vi "Gyro.vi"(8 "error in (no error)":errorcluster, 11 "GyroDevRef":T1) -> (1 "Boolean":bool)   [LabVIEW 2013]
uses:
  <vilib>/Rock Robotics/WPI/Gyro/WPI_GyroDevRef.ctl
  <vilib>/Rock Robotics/SystemInterfaces/Typedef/FPGA_TypedefAnalogModule.ctl
  <vilib>/Rock Robotics/SystemInterfaces/AI/FPGA_AIChannel.ctl
  <vilib>/Rock Robotics/WPI/DriverStation/DriverStationLCD/WPI_DriverStationLCDLCDLine.ctl
  Robot Global Data.vi
  <vilib>/Rock Robotics/WPI/Joystick/WPI_JoystickGetSetRefNum.vi
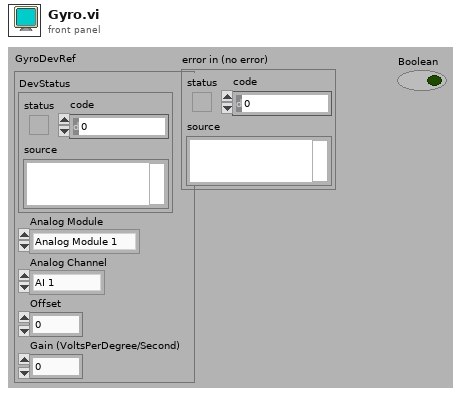
[diagram p1: front panel]
types:
  T1 = typedef "WPI_GyroDevRef.ctl" = cluster{"DevStatus":errorcluster, "Analog Module":T2, "Analog Channel":T3, "Offset":dbl, "Gain (VoltsPerDegree/Second)":dbl}
  T2 = typedef "FPGA_TypedefAnalogModule.ctl" = enum16{"Analog Module 1", "Analog Module 2"}
  T3 = typedef "FPGA_AIChannel.ctl" = enum8{"AI 1", "AI 2", "AI 3", "AI 4", "AI 5", "AI 6", "AI 7", "AI 8", "Invalid"}
  T4 = typedef "WPI_DriverStationLCDLCDLine.ctl" = enum16{"Main - Line 1", "User - Line 2", "User - Line 3", "User - Line 4", "User - Line 5", "User - Line 6"}
  T5 = typedef "WPI_JoystickDevRef.ctl" = cluster{"Device":T6}
  T6 = typedef "WPI_JoystickDeviceEnum.ctl" = enum16{"USB 1", "USB 2", "USB 3", "USB 4", "Kinect 1", "Kinect 2"}
  T7 = cluster{"axis 1 (x)":dbl, "axis 2 (y)":dbl, "axis 3 (throttle)":dbl, "axis 4":dbl, "axis 5":dbl, "axis 6":dbl}
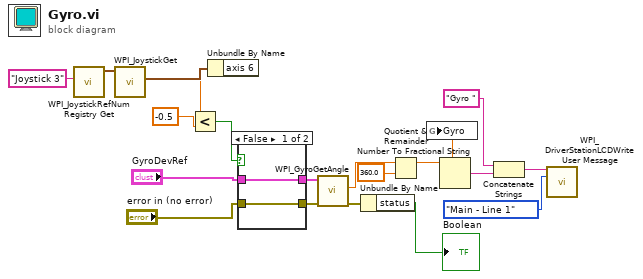
[diagram p0: block diagram]
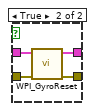
[diagram p2: hidden frame]
diagram:
  n1 = call <vilib>:"WPI_JoystickRefNum Registry Get.vi"("refnum name"="Joystick 3") -> ("JoystickDevRef"=w6:T5)  [unwired: 1 in, 9 out]
  n2 = call <vilib>:"WPI_JoystickGet.vi"("JoystickDevRef"=w6) -> ("Axes"=w5:T7)  [unwired: 1 in, 5 out]
  n3 = Unbundle By Name(w5) -> ("axis 6"=w3:dbl)
  n4 = Less?(x=w3, y=-0.5 ("x")) -> (x < y?=w4:bool)
  n5 = case shown="False" w4 {
    tunnel: [w21 w25] -> w14
    tunnel: [w20 w24] -> w11
    tunnel: "GyroDevRef" -> [w21 w23]
    tunnel: "error in (no error)" -> [w20 w22]
    frame False {
    }
    frame True {
      n6 = call <vilib>:"WPI_GyroReset.vi"("error in (no error)"=w22, "GyroDevRef"=w23) -> ("error out"=w24:errorcluster, "GyroDevRef"=w25:T1)  [unwired: 8 out]
    }
  }
  n7 = call <vilib>:"WPI_GyroGetAngle.vi"("error in (no error)"=w11, "GyroDevRef"=w14) -> ("error out"=w13:errorcluster, "Angle"=w18:dbl)  [unwired: 8 out]
  n8 = Unbundle By Name(w13) -> ("status"=→"Boolean":bool)
  n9 = Quotient & Remainder(x=w18, y=360.0) -> (x-y*floor(x/y)=w1:dbl)  [unwired: 1 out]
  n10 = global write "Robot Global Data.vi" "Gyro"(w1) -> ()
  n11 = Number To Fractional String(number=w1) -> (F-format string=w16:string)  [unwired: 3 out]
  n12 = Concatenate Strings("Gyro " ("string"), w16) -> (w12:string)
  n13 = call <vilib>:"WPI_DriverStationLCDWrite User Message.vi"("line text"=w12, "line"=WPI_DriverStationLCDLCDLine."Main - Line 1") -> ()  [unwired: 3 in, 11 out]
